vi "Serial Plotter 2 Values.vi"() -> ()   [LabVIEW 2014]
uses:
  <vilib>/Instr/_visa.llb/VISA Configure Serial Port (Instr).vi
panel:
  out "String":string="835,951\r\n"
  out "error IO":errorcluster
  in  "baud rate":u32=115200
  out "Waveform Chart":cluster{dbl, dbl}(graph)={835.0, 951.0}
  in  "stop":bool
  in  "COM port":refnum<visa-resource-name>="COM5"
  in  "error in":errorcluster
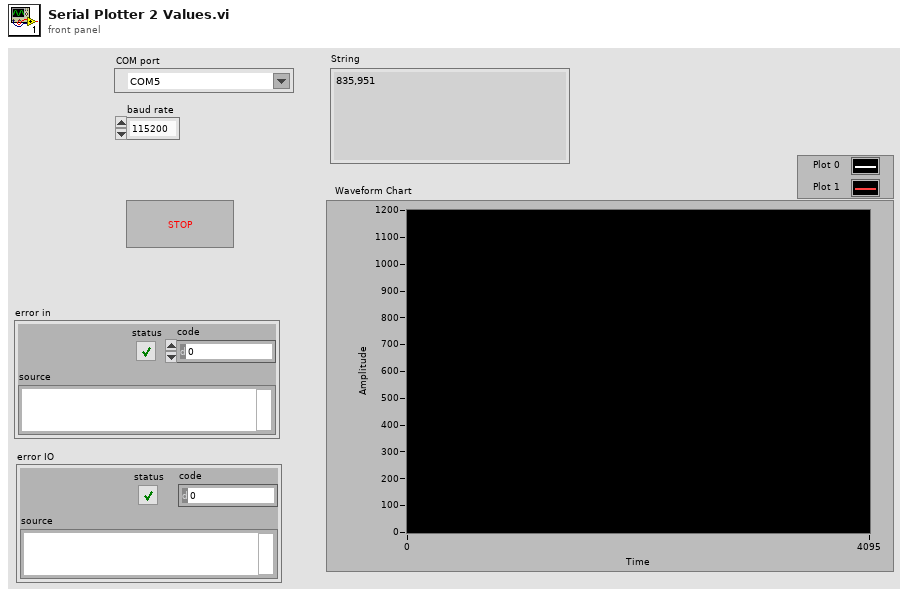
[diagram p1: front panel]
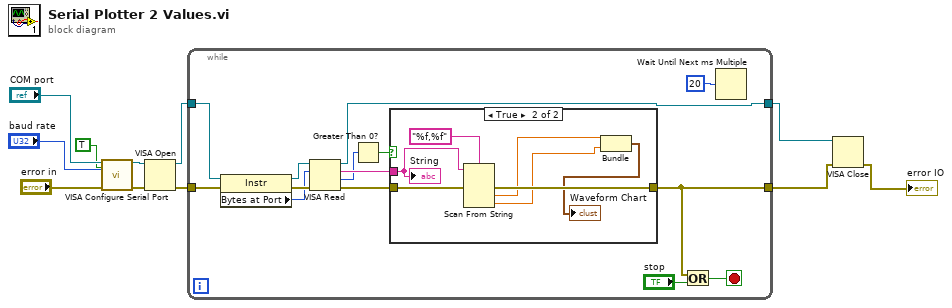
[diagram p0: block diagram]
diagram:
  n1 = call-poly "VISA Configure Serial Port"("VISA resource name"="COM port", "Enable Termination\nChar (T)"=TRUE ("Enable Termination\nChar (T)"), "baud rate (9600)"="baud rate", "error in (no error)"="error in") -> ("VISA resource name out"=w6:refnum<visa-resource-name>, "error out"=w8:errorcluster)  [unwired: 10 in]
  n2 = VISA Open(error in (no error)=w8, VISA resource name=w6) -> (VISA resource name=w10:refnum<visa-resource-name>, error out=w11:errorcluster)  [unwired: 3 in]
  n3 = while {
    tunnel: w11 -> [w21]
    tunnel: [w15] -> w3
    tunnel: w10 -> [w18]
    tunnel: [w12] -> w1
    stop <- w13 stop-if-true
    n4 = property class="Instr"(reference=w18, error in=w21) -> (reference out=w19:refnum<visa-resource-name>, error out=w20:errorcluster, "Bytes at Port"=w17:u32)
    n5 = VISA Read(VISA resource name=w19, byte count=w17, error in (no error)=w20) -> (VISA resource name out=w12:refnum<visa-resource-name>, read buffer=w25:string, return count=w22:u32, error out=w24:errorcluster)
    n6 = Greater Than 0?(x=w22) -> (x > 0?=w23:bool)
    n7 = case shown="True" w23 {
      tunnel: w25 -> [_ w30]
      tunnel: w24 -> [w26 w32]
      tunnel: [w26 w31] -> w15
      frame False {
      }
      frame True {
        n8 = Scan From String(format string="%f,%f", input string=w30, error in=w32) -> (error out=w31:errorcluster, output 1=w28:dbl, output 2=w29:dbl)  [unwired: 3 in, 2 out]
        n9 = Bundle(w28, w29) -> (→"Waveform Chart":cluster{dbl, dbl})  [unwired: 1 in]
        "String" <- w30
      }
    }
    n10 = Or(x=w15, y="stop") -> (x .or. y?=w13:bool)
    n11 = Wait Until Next ms Multiple(millisecond multiple=u32 20) -> ()  [unwired: 1 out]
  }
  n12 = VISA Close(VISA resource name=w1, error in (no error)=w3) -> (error out=→"error IO":errorcluster)
